vi "Separate Compiled Code From Source VIs.vi"() -> ()   [LabVIEW 2012]
doc: "Parses <b>Search Path</b> for <b>File Type</b> and sets the \"Separate compiled code from source file\" option. Saves all modified files."
panel:
  in  "File Type":string(combo)="*.vi"
  out "Removed":u32
  out "String":string
  out "Slide":u16(slide) caption="12/12" scale=-1.0..12.0
  out "error out":errorcluster
  out "All Files in Dir":path[](array[path])
  out "Array":errorcluster[](array[cluster])
  in  "Search Path":path
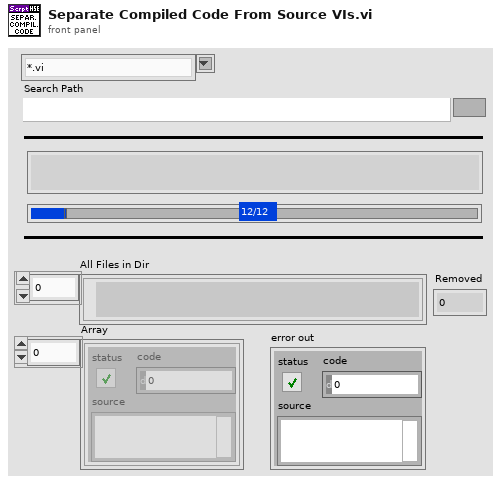
[diagram p1: front panel]
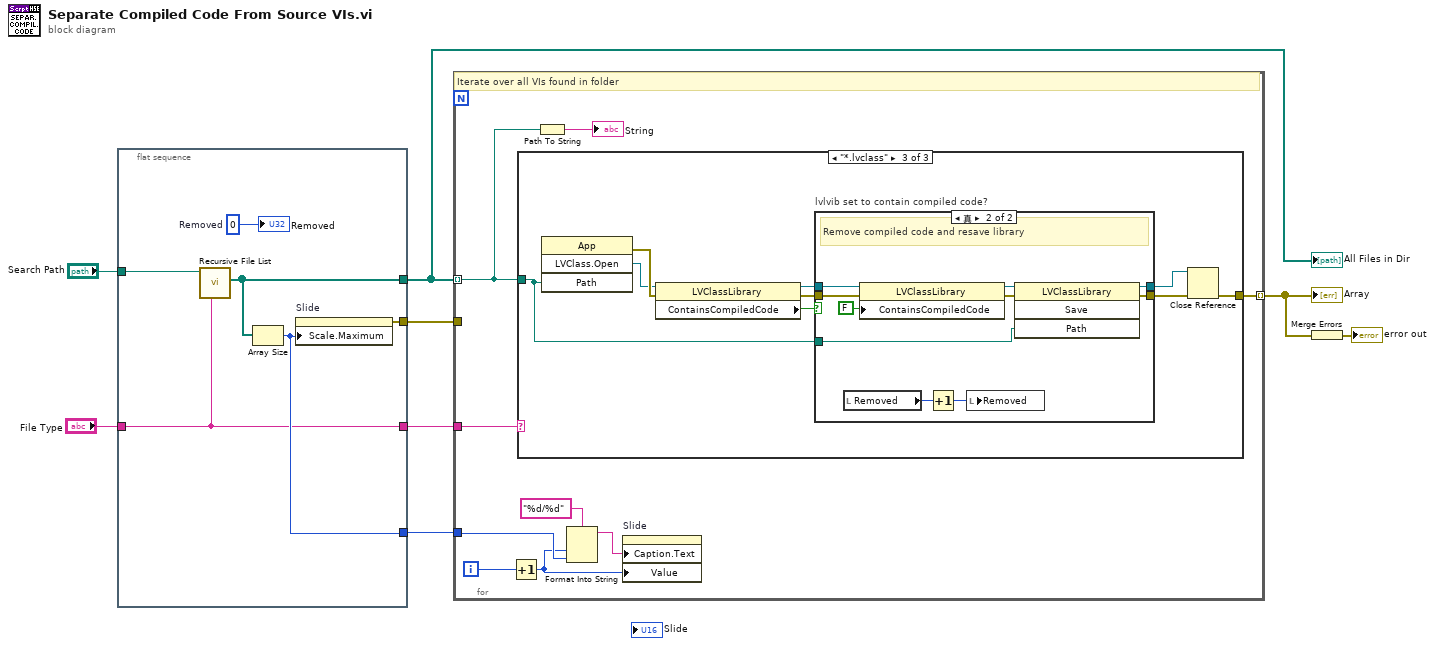
[diagram p0: block diagram]
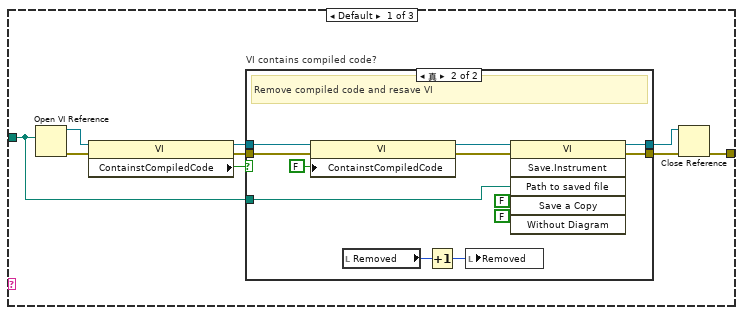
[diagram p2: hidden frame]
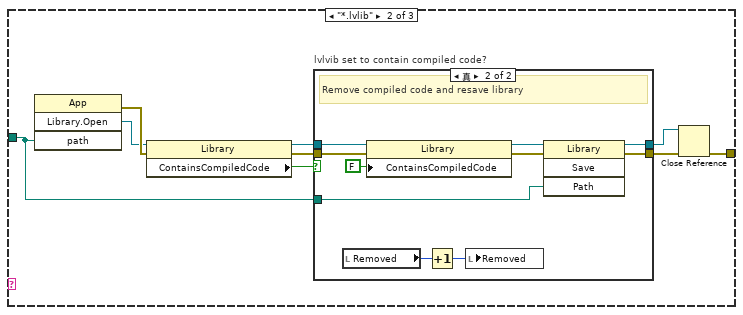
[diagram p4: hidden frame]
diagram:
  n1 = flat-sequence {
    tunnel: "Search Path" -> [w14]
    tunnel: [w13] -> w5
    tunnel: [w12] -> w4
    tunnel: [w11] -> w3
    tunnel: [w9] -> w2
    tunnel: "File Type" -> [w9]
    frame #0 {
      w10 = u32 0  # Removed
      n2 = call <vilib>:"Recursive File List.vi"("pattern"=w9, "Folder Path"=w14) -> ("All Files in Dir"=w13:path[])  [unwired: 5 in, 4 out]
      n3 = Array Size(array=w13) -> (size(s)=w11:i32)
      n4 = property on="Slide" class="Slide (严格)"("Scale.Maximum"=w11) -> (error out=w12:errorcluster)  [unwired: 2 in, 1 out]
      "Removed" <- w10
    }
  }
  n5 = for {
    tunnel: w5 -> [w16] mode=indexing
    tunnel: [w23] -> w7 mode=indexing
    tunnel: w4 -> [_]
    tunnel: w3 -> [w20]
    tunnel: w2 -> [w15]
    i -> [w21]
    # "Iterate over all VIs found in folder"
    n6 = Increment(x=w21) -> (x+1=w17:i32)
    n7 = case shown="\"*.lvclass\"" w15 {
      tunnel: [w30 w53 w74] -> w23
      tunnel: w16 -> [w24 w49 w70]
      frame Default {
        n8 = Open VI Reference(vi path=w24) -> (vi reference=w29:refnum<vi>, error out=w28:errorcluster)  [unwired: 5 in]
        n9 = property class="VI"(reference=w29, error in=w28) -> (reference out=w27:refnum<vi>, error out=w26:errorcluster, "ContainstCompiledCode"=w25:bool)
        n10 = case "VI contains compiled code?" shown="真" w25 {
          tunnel: [w34 w46] -> w32
          tunnel: [w33 w45] -> w31
          tunnel: w24 -> [_ w39]
          tunnel: w27 -> [w33 w38]
          tunnel: w26 -> [w34 w37]
          frame False {
            # "no compiled code - do nothing"
          }
          frame True {
            # "Remove compiled code and resave VI"
            n11 = property class="VI"(reference=w38, error in=w37, "ContainstCompiledCode"=FALSE ("Contains Compiled Code")) -> (reference out=w42:refnum<vi>, error out=w40:errorcluster)
            n12 = local read "Removed"() -> (w36:u32)
            n13 = Increment(x=w36) -> (x+1=w35:u32)
            n14 = local write "Removed"(w35) -> ()
            n15 = invoke class="VI" method="Save.Instrument"(reference=w42, error in=w40, "Path to saved file"=w39, "Save a Copy"=FALSE, "Without Diagram"=FALSE) -> (reference out=w45:refnum<vi>, error out=w46:errorcluster)  [unwired: 1 in, 4 out]
          }
        }
        n16 = Close Reference(reference=w31, error in (no error)=w32) -> (error out=w30:errorcluster)
      }
      frame "*.lvlib" {
        n17 = invoke class="App" method="Library.Open"("path"=w49) -> (error out=w48:errorcluster, "Open Library"=w47:refnum<vi>)  [unwired: 3 in, 2 out]
        n18 = property class="Library"(reference=w47, error in=w48) -> (reference out=w52:refnum<vi>, error out=w51:errorcluster, "ContainsCompiledCode"=w50:bool)
        n19 = case "lvlvib set to contain compiled code?" shown="真" w50 {
          tunnel: [w57 w67] -> w55
          tunnel: [w56 w66] -> w54
          tunnel: w49 -> [_ w62]
          tunnel: w52 -> [w56 w58]
          tunnel: w51 -> [w57 w61]
          frame False {
            # "no compiled code - do nothing"
          }
          frame True {
            # "Remove compiled code and resave library"
            n20 = local read "Removed"() -> (w60:u32)
            n21 = property class="Library"(reference=w58, error in=w61, "ContainsCompiledCode"=FALSE ("Contains Compiled Code")) -> (reference out=w65:refnum<vi>, error out=w63:errorcluster)
            n22 = Increment(x=w60) -> (x+1=w59:u32)
            n23 = local write "Removed"(w59) -> ()
            n24 = invoke class="Library" method="Save"(reference=w65, error in=w63, "Path"=w62) -> (reference out=w66:refnum<vi>, error out=w67:errorcluster)  [unwired: 1 in, 2 out]
          }
        }
        n25 = Close Reference(reference=w54, error in (no error)=w55) -> (error out=w53:errorcluster)
      }
      frame "*.lvclass" {
        n26 = invoke class="App" method="LVClass.Open"("Path"=w70) -> (error out=w69:errorcluster, "LVClass.Open"=w68:refnum<vi>)  [unwired: 3 in, 2 out]
        n27 = property class="LVClassLibrary"(reference=w68, error in=w69) -> (reference out=w73:refnum<vi>, error out=w72:errorcluster, "ContainsCompiledCode"=w71:bool)
        n28 = case "lvlvib set to contain compiled code?" shown="真" w71 {
          tunnel: [w78 w88] -> w76
          tunnel: [w77 w87] -> w75
          tunnel: w70 -> [_ w83]
          tunnel: w73 -> [w77 w79]
          tunnel: w72 -> [w78 w82]
          frame False {
            # "no compiled code - do nothing"
          }
          frame True {
            # "Remove compiled code and resave library"
            n29 = local read "Removed"() -> (w81:u32)
            n30 = property class="LVClassLibrary"(reference=w79, error in=w82, "ContainsCompiledCode"=FALSE ("Contains Compiled Code")) -> (reference out=w86:refnum<vi>, error out=w84:errorcluster)
            n31 = Increment(x=w81) -> (x+1=w80:u32)
            n32 = local write "Removed"(w80) -> ()
            n33 = invoke class="LVClassLibrary" method="Save"(reference=w86, error in=w84, "Path"=w83) -> (reference out=w87:refnum<vi>, error out=w88:errorcluster)  [unwired: 1 in, 2 out]
          }
        }
        n34 = Close Reference(reference=w75, error in (no error)=w76) -> (error out=w74:errorcluster)
      }
    }
    n35 = Path To String(path=w16) -> (string=→"String":string)
    n36 = Format Into String(format string="%d/%d", w17, w20) -> (resulting string=w18:string)  [unwired: 2 in, 1 out]
    n37 = property on="Slide" class="Slide (严格)"("Caption.Text"=w18, "Value"=w17) -> ()  [unwired: 2 in, 2 out]
  }
  "Array" <- w7
  n38 = Merge Errors(w7) -> (→"error out":errorcluster)
  "All Files in Dir" <- w5
